vi "Lockin Engine.vi"(8 "error in (no error)":errorcluster, 10 "Signal in":waveform(dbl)[](array[waveform]), 11 "lockin config":T1 {"TC (s)" format="%#_13g"}) -> (0 "error out":errorcluster, 2 "Lockin Results":T2)   [LabVIEW 2016, in "DSP.lockin.lvclass"]
uses:
  DSP.lockin.lvclass
  Typedefs/LockinResults.ctl
  Typedefs/LockinResult.ctl
  Typedefs/Lockin_Config.ctl
  <vilib>/Analysis/baseanly.llb/Mean (DBL).vi
  <vilib>/Analysis/NI_AALBase.lvlib
panel:
  out "filter fC (Hz)":dbl=0.3183098861837907
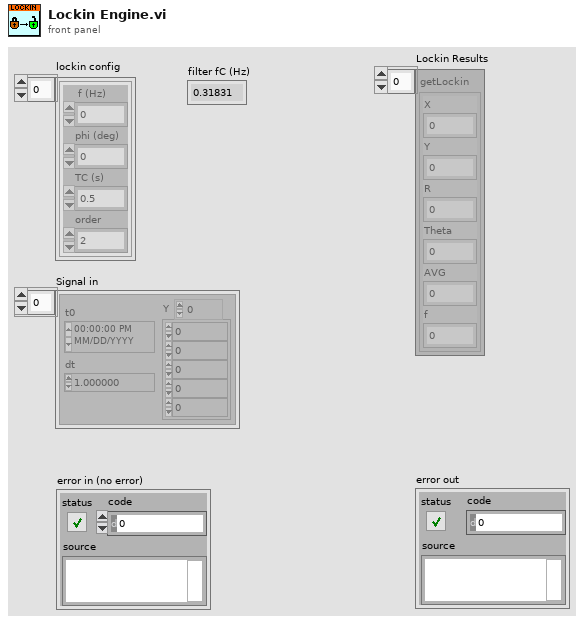
[diagram p1: front panel]
types:
  T1 = typedef "DSP.lockin.lvclass/Lockin_Config.ctl" = cluster{" f (Hz)":dbl, "phi (deg)":dbl, "TC (s)":dbl, "order":i32}[]
  T2 = typedef "DSP.lockin.lvclass/LockinResults.ctl" = T3[]
  T3 = typedef "DSP.lockin.lvclass/LockinResult.ctl" = cluster{"X":dbl, "Y":dbl, "R":dbl, "Theta":dbl, "AVG":dbl, "f":dbl}
  T4 = cluster{" f (Hz)":dbl, "phi (deg)":dbl, "TC (s)":dbl, "order":i32}
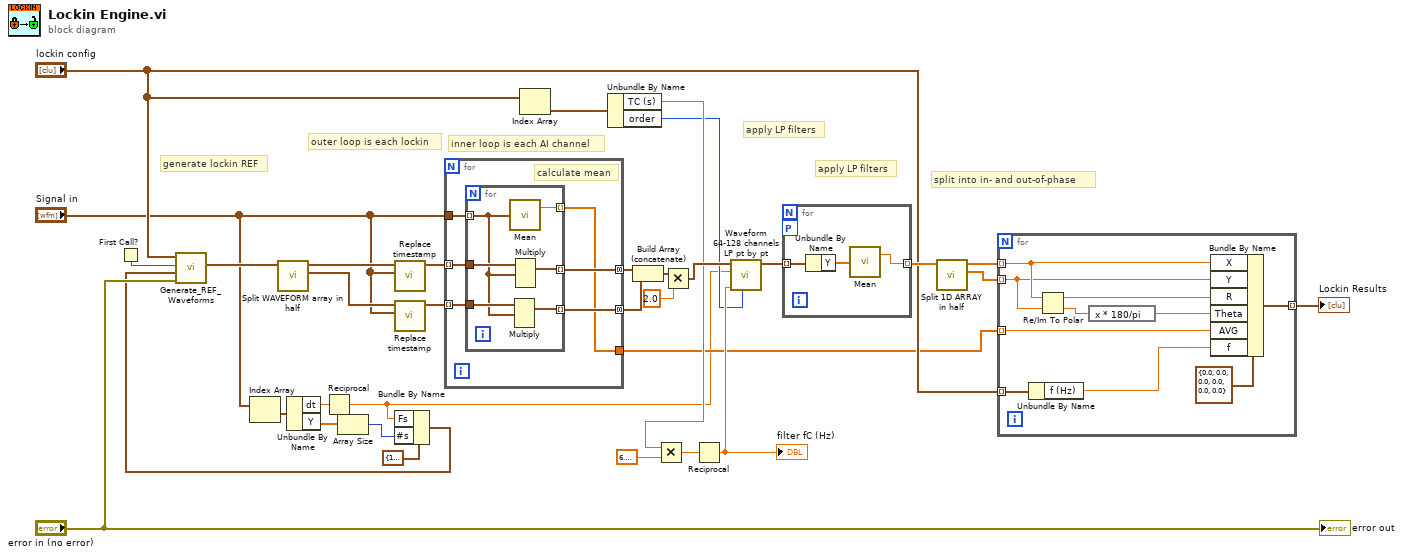
[diagram p0: block diagram]
diagram:
  # "generate lockin REF"
  # "split into in- and out-of-phase"
  # "apply LP filters"
  # "apply LP filters"
  # "inner loop is each AI channel"
  # "outer loop is each lockin"
  n1 = First Call?() -> (First Call?: T/F=w11:bool)
  n2 = Index Array(array="Signal in") -> (element=w17:waveform(dbl))  [unwired: 1 in]
  n3 = Unbundle By Name(w17) -> ("dt"=w16:dbl, "Y"=w14:dbl[])
  n4 = Reciprocal(x=w16) -> (1/x=w1:dbl)
  n5 = Array Size(array=w14) -> (size(s)=w12:i32)
  n6 = Bundle By Name(cluster=cluster{"Fs":dbl, "#s":dbl} {"Fs"=1000.0, "#s"=1000.0} ("sampling info"), "Fs"=w1, "#s"=w12) -> (w4:cluster{"Fs":dbl, "#s":dbl})
  n7 = call "Generate_REF_Waveforms.vi"("error in (no error)"="error in (no error)", "sampling info"=w4, "reset signal"=w11, "lockin config"="lockin config") -> ("REF Waveforms"=w15:waveform(dbl)[])  [unwired: 6 in, 1 out]
  n8 = call "Split WAVEFORM array in half.vi"("AO Array"=w15) -> ("Array 2"=w26:waveform(dbl)[], "Array 1"=w25:waveform(dbl)[])  [unwired: 9 in]
  n9 = call "Replace timestamp.vi"("Array 2"="Signal in", "Array 1"=w25) -> ("Array Out"=w28:waveform(dbl)[])  [unwired: 9 in]
  n10 = call "Replace timestamp.vi"("Array 2"="Signal in", "Array 1"=w26) -> ("Array Out"=w27:waveform(dbl)[])  [unwired: 9 in]
  n11 = for {
    tunnel: [w39] -> w22 mode=concatenating
    tunnel: [w38] -> w23 mode=concatenating
    tunnel: w27 -> [w37] mode=indexing
    tunnel: w28 -> [w36] mode=indexing
    tunnel: "Signal in" -> [w35]
    tunnel: [w34] -> w2
    # "calculate mean"
    n12 = for {
      tunnel: [w45] -> w38 mode=indexing
      tunnel: w37 -> [w42]
      tunnel: w35 -> [w41] mode=indexing
      tunnel: w36 -> [w43]
      tunnel: [w44] -> w39 mode=indexing
      tunnel: [w40] -> w34 mode=indexing
      n13 = Multiply(1:w41, 2:w42) -> (0:w45:waveform(dbl))  [unwired: 1 in, 1 out]
      n14 = call-poly <vilib>:"Mean.vi"("X"=w41) -> ("mean"=w40:dbl)  [unwired: 1 out]
      n15 = Multiply(1:w41, 2:w43) -> (0:w44:waveform(dbl))  [unwired: 1 in, 1 out]
    }
  }
  n16 = Index Array(array="lockin config") -> (element=w10:T4)  [unwired: 1 in]
  n17 = Unbundle By Name(w10) -> ("TC (s)"=w9:dbl, "order"=w8:i32)
  n18 = Build Array (concatenate)(w22, w23) -> (w24:waveform(dbl)[])
  n19 = Multiply(x=w9, y=6.283185307179586) -> (x*y=w21:dbl)
  n20 = Multiply(x=w24, y=2.0) -> (x*y=w33:waveform(dbl)[])
  n21 = Reciprocal(x=w21) -> (1/x=w29:dbl)
  "filter fC (Hz)" <- w29
  n22 = call "Waveform 64-128 channels LP pt by pt.vi"("order"=w8, "fl"=w29, "fs"=w1, "Array in"=w33) -> ("Array out"=w30:waveform(dbl)[])  [unwired: 7 in]
  n23 = for {
    tunnel: [w47] -> w31 mode=indexing
    workers-P: _ -> [_]
    tunnel: w30 -> [w46] mode=indexing
    n24 = Unbundle By Name(w46) -> ("Y"=w48:dbl[])
    n25 = call-poly <vilib>:"Mean.vi"("X"=w48) -> ("mean"=w47:dbl)  [unwired: 1 out]
  }
  n26 = call "Split 1D ARRAY in half.vi"("Array in"=w31) -> ("Array out"=w19:dbl[], "Array 3"=w18:dbl[])  [unwired: 9 in]
  n27 = for {
    tunnel: w18 -> [w57] mode=indexing
    tunnel: w19 -> [w56] mode=indexing
    tunnel: "lockin config" -> [w53] mode=indexing
    tunnel: [w51] -> w7 mode=indexing
    tunnel: w2 -> [w49] mode=indexing
    n28 = Unbundle By Name(w53) -> ("f (Hz)"=w52:dbl)
    n29 = Re/Im To Polar(2:w56, 3:w57) -> (0:w58:dbl, 1:w55:dbl)
    n30 = expression code="x * 180/pi"(w58) -> (w54:dbl)
    n31 = Bundle By Name(cluster=T3 {"X"=0.0, "Y"=0.0, "R"=0.0, "Theta"=0.0, "AVG"=0.0, "f"=0.0} ("Lockin Result"), "X"=w57, "Y"=w56, "R"=w55, "Theta"=w54, "AVG"=w49, "f"=w52) -> (w51:T3)
  }
  "Lockin Results" <- w7
  "error out" <- "error in (no error)"
